vi "UnInit.vi"(2 "Container State":T1 caption="容器状态", 3 "Display State":T2={"Front Color"=1985280, "User Event"=refnum} caption="显示状态") -> ()   [LabVIEW 2013, in "IP Adresss Control.xctl"]
uses:
  IP Adresss Control.xctl
  IP Address Status.ctl
  UserEvent/IP User Event.ctl
  <vilib>/_xctls/Container State.ctl
  <vilib>/_xctls/XControlSupport.lvlib
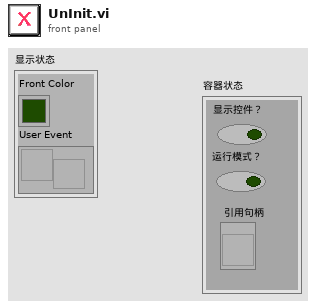
[diagram p1: front panel]
types:
  T1 = typedef "XControlSupport.lvlib/Container State.ctl" = cluster{"Indicator?":bool, "Run Mode?":bool, " Refnum":refnum<vi>}
  T2 = typedef "IP Adresss Control.xctl/IP Address Status.ctl" = cluster{"Front Color":u32, "User Event":refnum<user-event>}
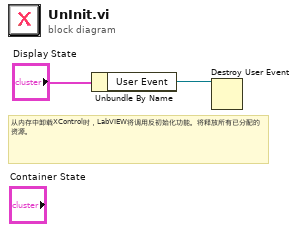
[diagram p0: block diagram]
diagram:
  # "从内存中卸载XControl时，LabVIEW将调用反初始化功能。将释放所有已分配的资源。"
  n1 = Unbundle By Name("Display State") -> ("User Event"=w1:refnum<user-event>)
  n2 = Destroy User Event(user event=w1) -> ()  [unwired: 1 in, 1 out]
